vi "Read DO_fnames.vi"(8 "error in (no error)":errorcluster, 11 "DO in":T1) -> (0 "error out":errorcluster, 2 "DO_fnames":string[](array[string]), 3 "DO out":T1)   [LabVIEW 2019, in "Inputs.lvlib"]
uses:
  Inputs.lvlib
  Ctl/DO.ctl
  Ctl/Parameter State.ctl
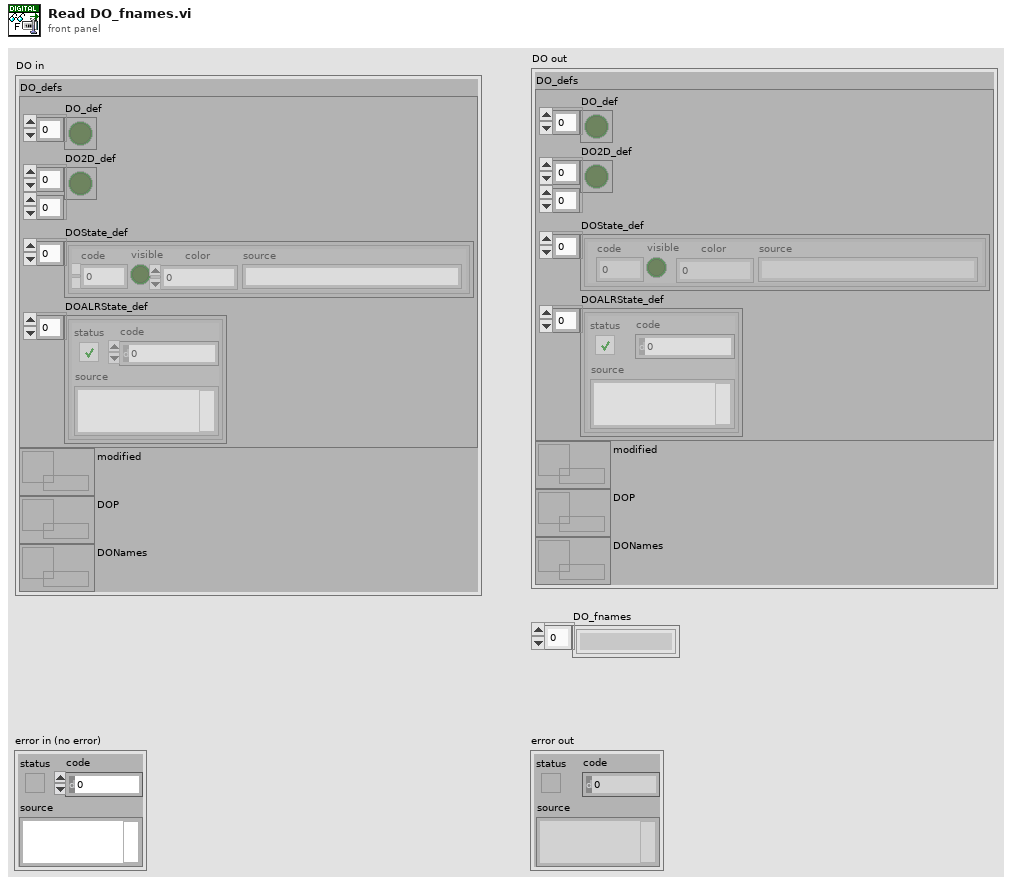
[diagram p1: front panel]
types:
  T1 = typedef "Inputs.lvlib/DO.ctl" = cluster{"DO_defs":cluster{"DO_def":bool[], "DO2D_def":bool[][], "DOState_def":T2[], "DOALRState_def":errorcluster[]}, "modified":refnum<data-value>, "DOP":refnum<data-value>, "DONames":refnum<data-value>}
  T2 = typedef "Inputs.lvlib/Parameter State.ctl" = cluster{"code":i32, "visible":bool, "color":u32, "source":string}
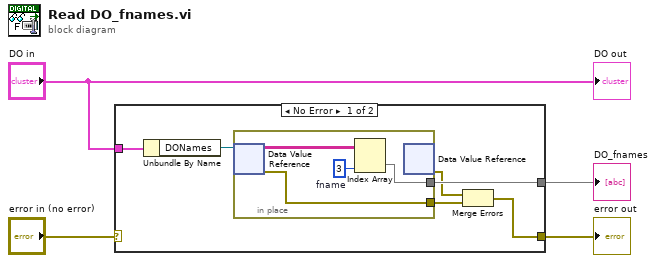
[diagram p0: block diagram]
diagram:
  n1 = case shown="No Error" "error in (no error)" {
    selector: "error in (no error)" -> [_ w15]
    tunnel: [w6 w15] -> w2
    tunnel: "DO in" -> [w5 _]
    tunnel: [w9 _] -> w3
    frame No Error {
      n2 = Unbundle By Name(w5) -> ("DONames"=w10:refnum<data-value>)
      n3 = in-place {
        in-place-border: [w14] -> w8
        in-place-border: [w11] -> w9
        w13 = 3  # fname
        n4 = in-place-dvr #1(w10) -> (w12:string[][], w14:errorcluster)
        n5 = Index Array(array=w12, index (col)=w13) -> (element=w11:string[])  [unwired: 1 in]
        n6 = in-place-dvr #1() -> (w7:errorcluster)  [unwired: 1 in, 1 out]
      }
      n7 = Merge Errors(w7, w8) -> (w6:errorcluster)
    }
    frame Error {
    }
  }
  "error out" <- w2
  "DO_fnames" <- w3
  "DO out" <- "DO in"
